vi "U3 Low Latency Stream.vi"() -> ()   [LabVIEW 2021]
panel:
  in  "# Channels":i32=4
  in  "Delay [ms]":u32
  out "Comm Backlog [%]":dbl format="%.2f"
  in  "Scans To Read Per Iteration":dbl=1.0 format="%.3f"
  out "UD Backlog [%]":dbl format="%.2f"
  out "Actual Scan Rate (Hz)":dbl format="%.3f"
  out "# Scans Read":i32
  out "# of iterations":i32
  out "Data":dbl[][](array[numeric]) format="%.3f"
  in  "Scan Rate (Hz)":dbl=10.0 format="%.3f"
  in  "stop":bool
  out "Error Message":string
  # "Usually command/response is used in low-latency applications.  Stream is good at collecting data fast at precise intervals,\nbut is most efficient when it moves large chunks of data at a time.  This VI demonstrates techniques for moving small\nchunks of data more often."
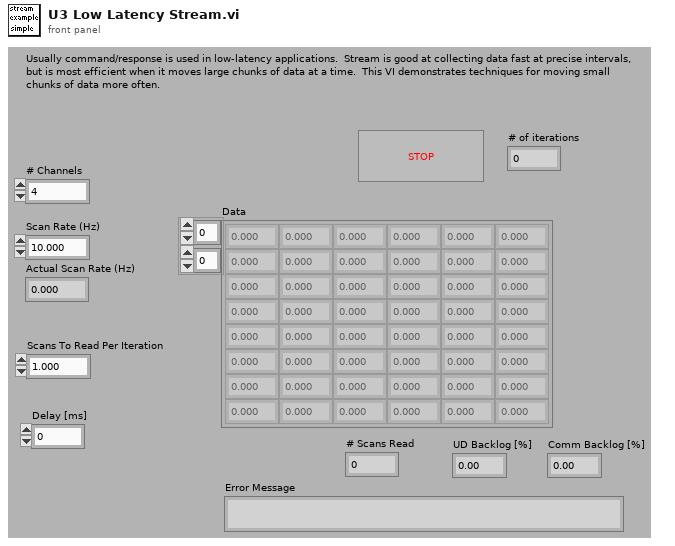
[diagram p1: front panel]
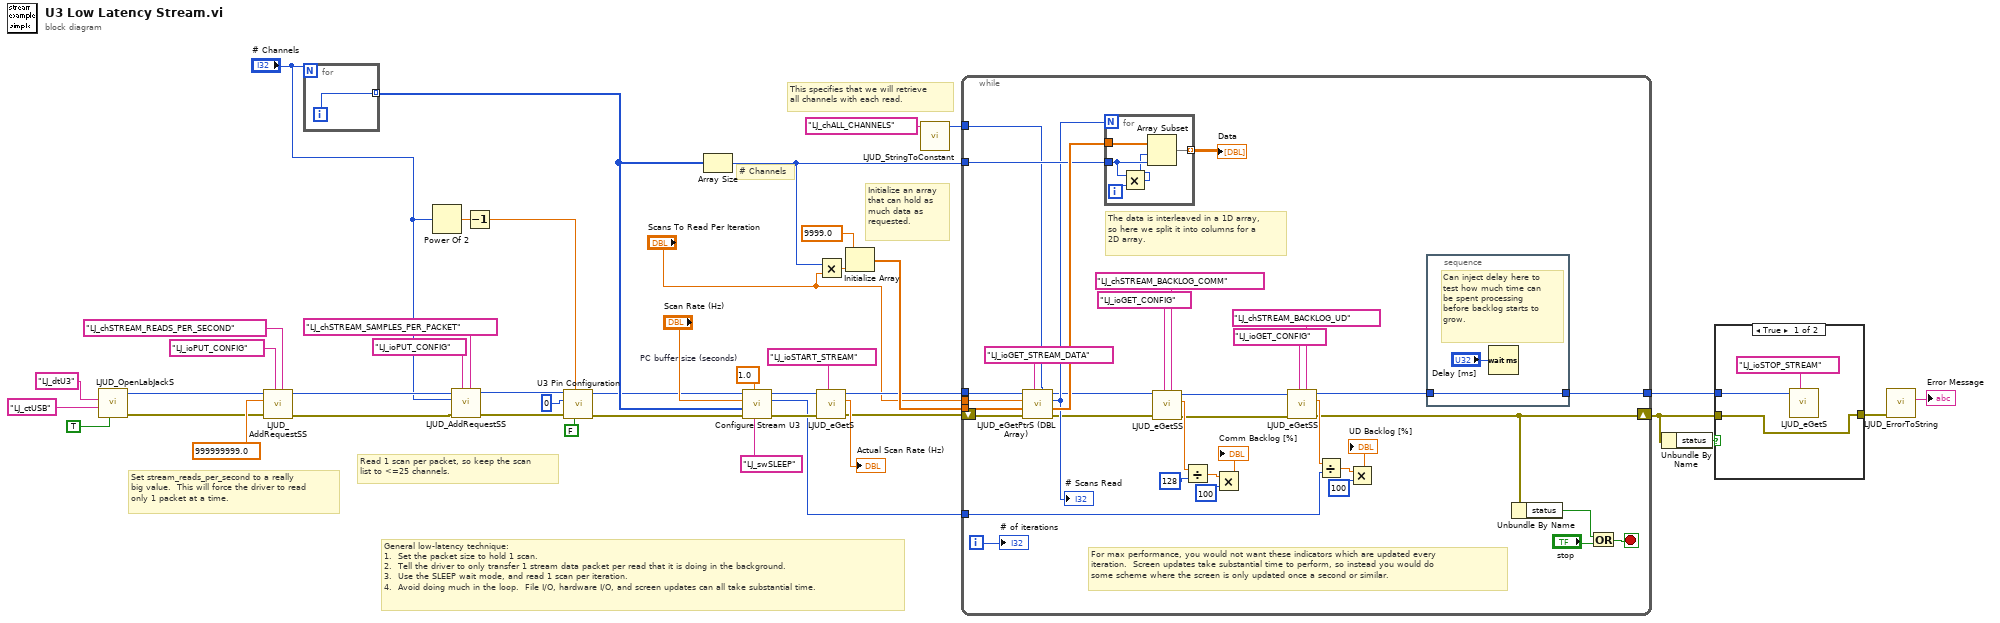
[diagram p0: block diagram]
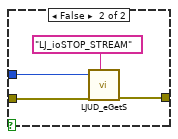
[diagram p2: hidden frame]
diagram:
  w11 = 1.0  # PC buffer size (seconds)
  # "General low-latency technique:\n1.  Set the packet size to hold 1 scan.\n2.  Tell the driver to only transfer 1 stream data packet per read that it is doing in the background.\n3.  Use the SLEEP wait mode, and read 1 scan per iteration.\n4.  Avoid doing much in the loop.  File I/O, hardware I/O, and screen updates can all take substantial time."
  # "Set stream_reads_per_second to a really\nbig value.  This will force the driver to read\nonly 1 packet at a time."
  # "Read 1 scan per packet, so keep the scan\nlist to <=25 channels."
  # "Initialize an array\nthat can hold as\nmuch data as\nrequested."
  # "# Channels"
  # "This specifies that we will retrieve\nall channels with each read."
  n1 = call "LJUD_OpenLabJackS.vi"("FirstFound"=TRUE, "ConnectionType"="LJ_ctUSB", "DeviceType"="LJ_dtU3") -> ("error out"=w14:errorcluster, "Handle"=w16:i32)  [unwired: 6 in, 1 out]
  n2 = call "LJUD_AddRequestSS.vi"("Channel"="LJ_chSTREAM_READS_PER_SECOND" ("IOType"), "IOType"="LJ_ioPUT_CONFIG", "error in"=w14, "Value"=999999999.0, "Handle In"=w16) -> ("error out"=w13:errorcluster, "Handle Out"=w15:i32)  [unwired: 5 in]
  n3 = for {
    N: "# Channels" -> [_]
    tunnel: [w45] -> w10 mode=indexing
    i -> [w45]
  }
  n4 = Power Of 2(x="# Channels") -> (2^x=w2:dbl)
  n5 = call "LJUD_AddRequestSS.vi"("Channel"="LJ_chSTREAM_SAMPLES_PER_PACKET" ("IOType"), "IOType"="LJ_ioPUT_CONFIG", "error in"=w13, "Value"="# Channels", "Handle In"=w15) -> ("error out"=w9:errorcluster, "Handle Out"=w7:i32)  [unwired: 5 in]
  n6 = Decrement(x=w2) -> (x-1=w1:dbl)
  n7 = call "U3 Pin Configuration.vi"("Enable Counter0"=FALSE, "FIO/EIO Analog Enable"=w1, "error in"=w9, "Number of Timers Enabled"=u8 0, "Handle In"=w7) -> ("error out"=w8:errorcluster, "Handle Out"=w6:i32)  [unwired: 5 in]
  n8 = Array Size(array=w10) -> (size(s)=w38:i32)
  n9 = call "Configure Stream U3.vi"("Wait Mode"="LJ_swSLEEP" ("Wait Mode (2)"), "PC buffer size (seconds)"=w11, "error in"=w8, "Scan List (+)"=w10, "Scan Rate (Hz)"="Scan Rate (Hz)", "Handle In"=w6) -> ("error out"=w42:errorcluster, "PC buffer size (samples)"=w24:i32, "Handle Out"=w43:i32)  [unwired: 3 in]
  n10 = Multiply(x=w38, y="Scans To Read Per Iteration") -> (x*y=w41:dbl)
  n11 = call "LJUD_eGetS.vi"("IOType"="LJ_ioSTART_STREAM", "error in"=w42, "Handle In"=w43) -> ("error out"=w27:errorcluster, "Value Read"=→"Actual Scan Rate (Hz)":dbl, "Handle Out"=w32:i32)  [unwired: 6 in]
  n12 = Initialize Array(9999.0, w41) -> (w39:dbl[])
  n13 = call "LJUD_StringToConstant.vi"("String"="LJ_chALL_CHANNELS") -> ("Constant Number"=w29:i32)  [unwired: 9 in, 1 out]
  n14 = while {
    tunnel: w24 -> [w59]
    shift-left: w27 -> [w67]
    shift-right: [w60] -> w28
    tunnel: w29 -> [w70]
    tunnel: [w57] -> w36
    tunnel: w38 -> [w73]
    tunnel: w39 -> [w76]
    tunnel: "Scans To Read Per Iteration" -> [w74]
    tunnel: w32 -> [w78]
    i -> [w72]
    stop <- w69 stop-if-true
    # "For max performance, you would not want these indicators which are updated every\niteration.  Screen updates take substantial time to perform, so instead you would do\nsome scheme where the screen is only updated once a second or similar."
    # "The data is interleaved in a 1D array,\nso here we split it into columns for a\n2D array."
    n15 = call "LJUD_eGetPtrS (DBL Array).vi"("Channel"=w70, "IOType"="LJ_ioGET_STREAM_DATA", "error in"=w67, "DBL Array Write"=w76, "Value"=w74, "Handle In"=w78) -> ("error out"=w48:errorcluster, "DBL Array Read"=w75:dbl[], "Value"=w68:i32, "Handle Out"=w47:i32)  [unwired: 2 in]
    "# Scans Read" <- w68
    n16 = for {
      N: w68 -> [_]
      tunnel: w75 -> [w87]
      tunnel: w73 -> [w86]
      tunnel: [w83] -> w71 mode=indexing
      i -> [w85]
      n17 = Multiply(x=w86, y=w85) -> (x*y=w84:i32)
      n18 = Array Subset(array=w87, index=w84, length=w86) -> (w83:dbl[])
    }
    "Data" <- w71
    n19 = call "LJUD_eGetSS.vi"("Channel"="LJ_chSTREAM_BACKLOG_COMM", "IOType"="LJ_ioGET_CONFIG", "error in"=w48, "Handle In"=w47) -> ("error out"=w49:errorcluster, "Value Read"=w56:dbl, "Handle Out"=w50:i32)  [unwired: 5 in]
    n20 = Divide(x=w56, y=128) -> (x/y=w53:dbl)
    n21 = Multiply(x=w53, y=100) -> (x*y=→"Comm Backlog [%]":dbl)
    n22 = call "LJUD_eGetSS.vi"("Channel"="LJ_chSTREAM_BACKLOG_UD", "IOType"="LJ_ioGET_CONFIG", "error in"=w49, "Handle In"=w50) -> ("error out"=w60:errorcluster, "Value Read"=w62:dbl, "Handle Out"=w58:i32)  [unwired: 5 in]
    n23 = Divide(x=w62, y=w59) -> (x/y=w63:dbl)
    n24 = Multiply(x=w63, y=100) -> (x*y=→"UD Backlog [%]":dbl)
    n25 = stacked-sequence {
      tunnel: w58 -> [w82]
      tunnel: [w82] -> w57
      frame #0 {
        # "Can inject delay here to\ntest how much time can\nbe spent processing\nbefore backlog starts to\ngrow."
        n26 = Wait (ms)(milliseconds to wait="Delay [ms]") -> ()  [unwired: 1 out]
      }
    }
    n27 = Unbundle By Name(w60) -> ("status"=w79:bool)
    n28 = Or(x=w79, y="stop") -> (x .or. y?=w69:bool)
    "# of iterations" <- w72
  }
  n29 = Unbundle By Name(w28) -> ("status"=w31:bool)
  n30 = case shown="True" w31 {
    tunnel: w36 -> [w89 w93]
    tunnel: [w88 w92] -> w35
    tunnel: w28 -> [w88 w91]
    frame True {
      n31 = call "LJUD_eGetS.vi"("IOType"="LJ_ioSTOP_STREAM", "Handle In"=w89) -> ()  [unwired: 7 in, 3 out]
    }
    frame False {
      n32 = call "LJUD_eGetS.vi"("IOType"="LJ_ioSTOP_STREAM", "error in"=w91, "Handle In"=w93) -> ("error out"=w92:errorcluster)  [unwired: 6 in, 2 out]
    }
  }
  n33 = call "LJUD_ErrorToString.vi"("error in"=w35) -> ("String"=→"Error Message":string)  [unwired: 10 in]
